vi "updateWaveform.vi"(8 "error in (no error)":errorcluster, 11 "Model in":refnum<class "Model.lvclass">) -> (0 "error out":errorcluster, 3 "Model out":refnum<class "Model.lvclass">)   [LabVIEW 2015, in "Model.lvclass"]
uses:
  Model.lvclass
  Model.lvclass/Model.ctl
  Waveforms/IWaveforms/IWaveform.lvclass
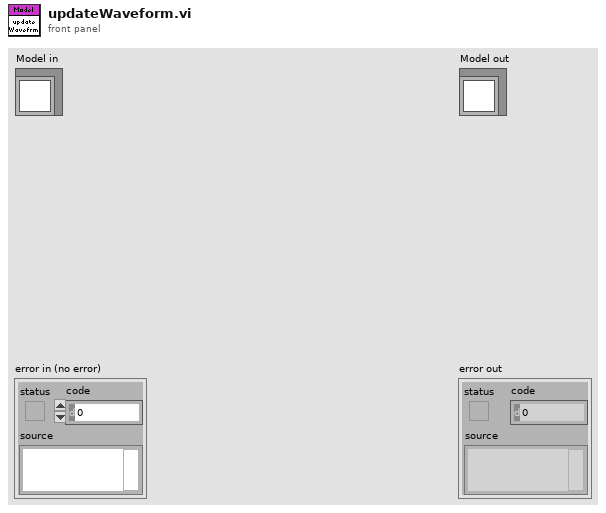
[diagram p1: front panel]
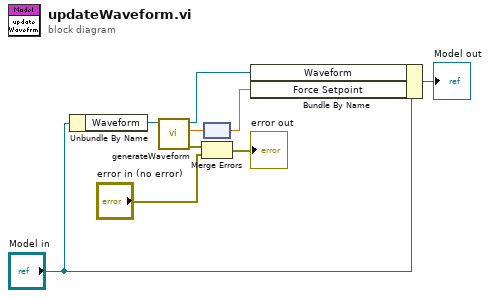
[diagram p0: block diagram]
diagram:
  n1 = Unbundle By Name("Model in") -> ("Waveform"=w7:refnum<class "IWaveform.lvclass">)
  n2 = call-dynamic "generateWaveform.vi"("IWaveform in"=w7) -> ("error out"=w3:errorcluster, "Output"=w5:dbl, "IWaveform out"=w6:refnum<class "IWaveform.lvclass">)  [unwired: 8 in]
  n3 = Merge Errors(w3, "error in (no error)") -> (→"error out":errorcluster)
  n4 = node(w5) -> (w4:dbl[unit])
  n5 = Bundle By Name(cluster="Model in", "Waveform"=w6, "Force Setpoint"=w4) -> (→"Model out":refnum<class "Model.lvclass">)
